vi "Scale and Unscale Test.vi"() -> ()   [LabVIEW 2016]
uses:
  Frames & Messages/TypeDefs/Scaling Information.ctl
  BCI-1553 API.lvlib
panel:
  out "Raw Value":u64 format="%016x"
  out "Scaled Value":dbl
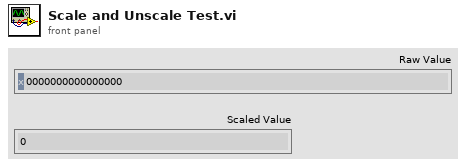
[diagram p1: front panel]
types:
  T1 = typedef "BCI-1553 API.lvlib/Scaling Information.ctl" = cluster{"Bit Offset":i32, "Bit Count":i32, "LSB Resolution":dbl, "2's Complement":bool, "Big Endian":bool, "Sign Bit":bool}
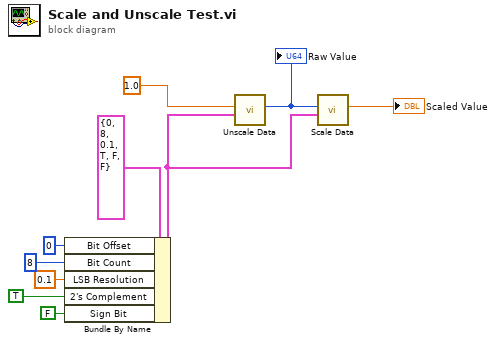
[diagram p0: block diagram]
diagram:
  n1 = Bundle By Name(cluster=T1 {"Bit Offset"=0, "Bit Count"=8, "LSB Resolution"=0.1, "2's Complement"=TRUE, "Big Endian"=FALSE, "Sign Bit"=FALSE} ("Scaling Info"), "Bit Offset"=0, "Bit Count"=8, "LSB Resolution"=0.1, "2's Complement"=TRUE, "Sign Bit"=FALSE) -> (w6:T1)
  n2 = call "Unscale Data.vi"("Scaling Info"=w6, "Scaled Value"=1.0) -> ("Raw Value"=w10:u64)  [unwired: 8 in, 1 out]
  "Raw Value" <- w10
  n3 = call "Scale Data.vi"("Scaling Info"=w6, "Raw Value"=w10) -> ("Scaled Value"=→"Scaled Value":dbl)  [unwired: 8 in, 1 out]
